vi "Configure Setpoint and Ramp.vi"(0 "VISA resource name":refnum<visa-resource-name>, 1 "Enable Setpoint Ramping  (F: Disable)":bool, 2 "Ramp Rate (0.0)":dbl format="%.3f", 5 "Output's Control Loop (1:1)":u16(ring)=1 items=["1"=1, "2"=2, "3"=3, "4"=4], 7 "Setpoint (0.00000)":dbl format="%.5f", 11 "error in (no error)":errorcluster) -> (4 "VISA resource name out":refnum<visa-resource-name>, 15 "error out":errorcluster)   [LabVIEW 2015, in "Lake Shore 350.lvlib"]
doc: "Configures the Setpoint and Setpoint Ramping function. The Setpoint parameter is used to set the desired load temperature for a control loop."
uses:
  Lake Shore 350.lvlib
  Instance           2 35Saved   Configure Setpoint and Ramp .vi
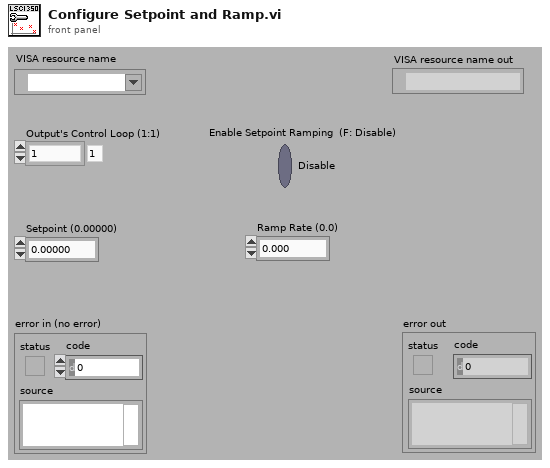
[diagram p1: front panel]
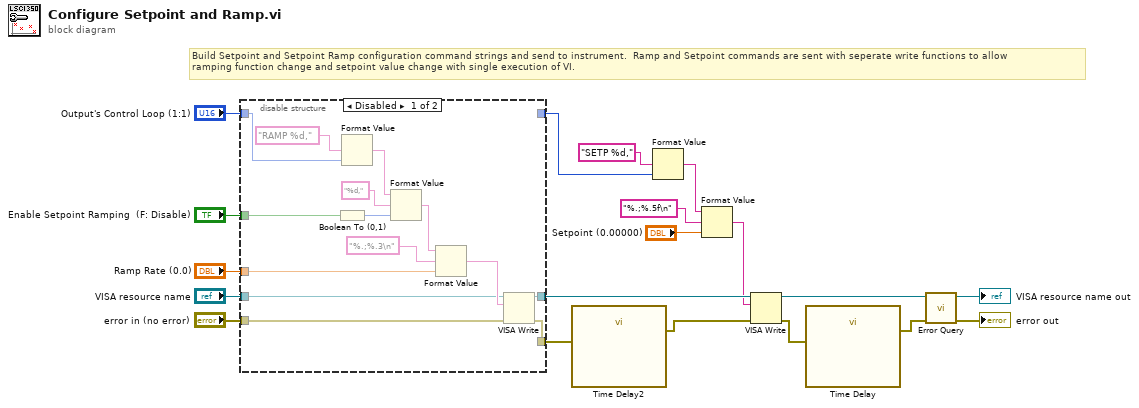
[diagram p0: block diagram]
diagram:
  # "Build Setpoint and Setpoint Ramp configuration command strings and send to instrument.  Ramp and Setpoint commands are sent with seperate write functions to allow\nramping function change and setpoint value change with single execution of VI."
  n1 = disable-structure shown="Disabled" {
    disable-tunnel: "Enable Setpoint Ramping  (F: Disable)" -> [w31 _]
    disable-tunnel: "Ramp Rate (0.0)" -> [w29 _]
    disable-tunnel: "Output's Control Loop (1:1)" -> [w25 w36]
    disable-tunnel: [w23 w35] -> w7
    disable-tunnel: [w22 w34] -> w6
    disable-tunnel: "VISA resource name" -> [w21 w35]
    disable-tunnel: "error in (no error)" -> [w20 w34]
    disable-tunnel: [_ w36] -> w1
    frame Disabled {
      n2 = Boolean To (0,1)(Boolean=w31) -> (0, 1=w32:i16)
      n3 = Format Value(format string="RAMP %d,", value (0)=w25) -> (output string=w26:string)  [unwired: 1 in]
      n4 = Format Value(string ("")=w26, format string="%d,", value (0)=w32) -> (output string=w30:string)
      n5 = Format Value(string ("")=w30, format string="%.;%.3\n", value (0)=w29) -> (output string=w24:string)
      n6 = VISA Write(VISA resource name=w21, write buffer=w24, error in (no error)=w20) -> (VISA resource name out=w23:refnum<visa-resource-name>, error out=w22:errorcluster)  [unwired: 1 out]
    }
    frame Enabled {
    }
  }
  n7 = call "Time Delay2"("error in (no error)"=w6) -> ("error out"=w5:errorcluster)  [unwired: 10 in]
  n8 = Format Value(format string="SETP %d,", value (0)=w1) -> (output string=w11:string)  [unwired: 1 in]
  n9 = Format Value(string ("")=w11, format string="%.;%.5f\n", value (0)="Setpoint (0.00000)") -> (output string=w4:string)
  n10 = VISA Write(VISA resource name=w7, write buffer=w4, error in (no error)=w5) -> (VISA resource name out=w19:refnum<visa-resource-name>, error out=w16:errorcluster)  [unwired: 1 out]
  n11 = call "Time Delay"("error in (no error)"=w16) -> ("error out"=w15:errorcluster)  [unwired: 10 in]
  n12 = call "Error Query.vi"("error in (no error)"=w15, "VISA resource name"=w19) -> ("error out"=→"error out":errorcluster, "VISA resource name out"=→"VISA resource name out":refnum<visa-resource-name>)  [unwired: 7 in, 1 out]
